vi "Write to TDMS(SubVI).vi"(8 "error in (no error)":errorcluster, 9 "LED state":string, 10 "element":T1 {"RMS" format="%0.6f"; "RPM" format="%0.2f"; "Voltage" format="%0.2f"; "Current" format="%0.2f"; "Temperature" format="%0.2f"}, 11 "Refnum in":refnum<k34>) -> (0 "error out":errorcluster, 3 "Refnum out":refnum<k34>)   [LabVIEW 2017]
uses:
  D:/Github/PTC-project.git/trunk/typedefs/Data.ctl
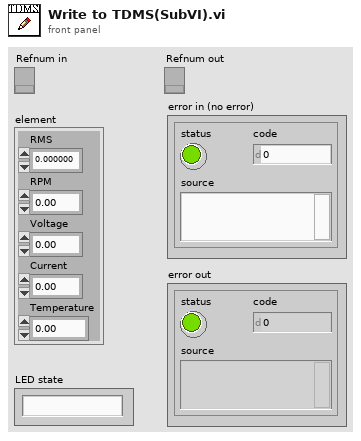
[diagram p1: front panel]
types:
  T1 = typedef "Data.ctl" = cluster{"RMS":dbl, "RPM":dbl, "Voltage":dbl, "Current":dbl, "Temperature":dbl}
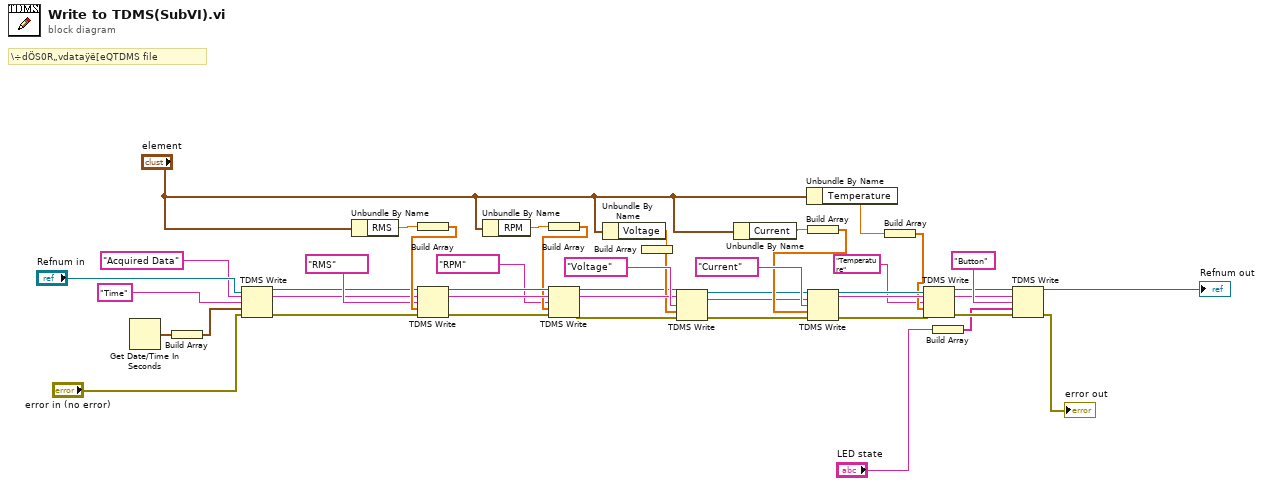
[diagram p0: block diagram]
diagram:
  # "\\÷dÖS0R„vdataÿë[eQTDMS file"
  n1 = Get Date/Time In Seconds() -> (seconds since 1Jan1904=w4:timestamp)
  n2 = Build Array(w4) -> (w5:timestamp[])
  n3 = TDMS Write(0:"Refnum in", 5:"Acquired Data" ("group name in (Untitled)"), 7:"Time" ("group name in (Untitled)"), 9:w5, 11:"error in (no error)") -> (4:w9:refnum<k34>, 6:w7:string, 15:w8:errorcluster)  [unwired: 1 in, 1 out]
  n4 = Unbundle By Name("element") -> ("RMS"=w10:dbl)
  n5 = Build Array(w10) -> (w12:dbl[])
  n6 = TDMS Write(0:w9, 5:w7, 7:"RMS" ("group name in (Untitled)"), 9:w12, 11:w8) -> (4:w15:refnum<k34>, 6:w16:string, 15:w17:errorcluster)  [unwired: 1 in, 1 out]
  n7 = Unbundle By Name("element") -> ("RPM"=w14:dbl)
  n8 = Build Array(w14) -> (w13:dbl[])
  n9 = TDMS Write(0:w15, 5:w16, 7:"RPM" ("group name in (Untitled)"), 9:w13, 11:w17) -> (4:w23:refnum<k34>, 6:w26:string, 15:w25:errorcluster)  [unwired: 1 in, 1 out]
  n10 = Unbundle By Name("element") -> ("Voltage"=w22:dbl)
  n11 = Build Array(w22) -> (w24:dbl[])
  n12 = TDMS Write(0:w23, 5:w26, 7:"Voltage" ("group name in (Untitled)"), 9:w24, 11:w25) -> (4:w20:refnum<k34>, 6:w19:string, 15:w18:errorcluster)  [unwired: 1 in, 1 out]
  n13 = Unbundle By Name("element") -> ("Current"=w21:dbl)
  n14 = Unbundle By Name("element") -> ("Temperature"=w32:dbl)
  n15 = Build Array(w21) -> (w28:dbl[])
  n16 = TDMS Write(0:w20, 5:w19, 7:"Current" ("group name in (Untitled)"), 9:w28, 11:w18) -> (4:w33:refnum<k34>, 6:w35:string, 15:w34:errorcluster)  [unwired: 1 in, 1 out]
  n17 = Build Array(w32) -> (w31:dbl[])
  n18 = TDMS Write(0:w33, 5:w35, 7:"Temperature" ("group name in (Untitled)"), 9:w31, 11:w34) -> (4:w38:refnum<k34>, 6:w37:string, 15:w42:errorcluster)  [unwired: 1 in, 1 out]
  n19 = Build Array("LED state") -> (w40:string[])
  n20 = TDMS Write(0:w38, 5:w37, 7:"Button" ("channel name(s) in (Untitled)"), 9:w40, 11:w42) -> (4:→"Refnum out":refnum<k34>, 15:→"error out":errorcluster)  [unwired: 1 in, 2 out]
